vi "Instrument Delay.vi"(5 "delay":dbl[unit] format="%.3f", 6 "error in":errorcluster, 9 "VISA resource":refnum<visa-resource-name>="GPIB0::9::INSTR") -> (0 "error out":errorcluster, 3 "VISA resource dup":refnum<visa-resource-name>)   [LabVIEW 2010]
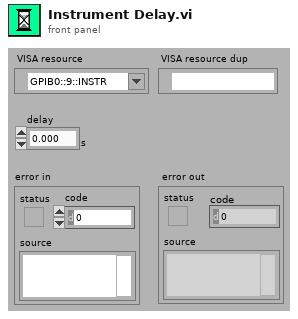
[diagram p1: front panel]
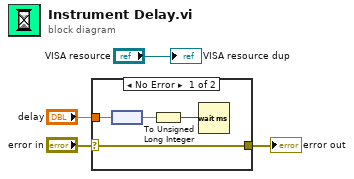
[diagram p0: block diagram]
diagram:
  n1 = case shown="No Error" "error in" {
    selector: "error in" -> [w5 w9]
    tunnel: "delay" -> [w8 _]
    tunnel: [w5 w9] -> w1
    frame No Error {
      n2 = node(w8) -> (w7:dbl)
      n3 = To Unsigned Long Integer(number=w7) -> (unsigned 32bit integer=w6:u32)
      n4 = Wait (ms)(milliseconds to wait=w6) -> ()  [unwired: 1 out]
    }
    frame Error {
    }
  }
  "error out" <- w1
  "VISA resource dup" <- "VISA resource"
